vi "Rotation3d_Equals.vi"(9 "other Rotation3d":T1={"Q_quaternion"={"R"=1.0, "V"=[0.0, 0.0, 0.0]}}, 11 "in Rotation3d":T1={"Q_quaternion"={"R"=1.0, "V"=[0.0, 0.0, 0.0]}}) -> (3 "Equals":bool)   [LabVIEW 2019, in "Trajectory_Library.lvlib"]
doc: "Checks equality between this Rotation3d and another object.\n\nParameters:\n\n - IN ROTATION3D -- This rotation3d data structure\n - OTHER ROTATION3D -- The rotation3d to compare.\n\nReturns:\n - Equals -- Returns TRUE if the two rotation3ds are equals."
uses:
  Trajectory_Library.lvlib
  TypeDef/ROTATION3D.ctl
  TypeDef/QUATERNION.ctl
  Quaternion_Get_Vect.vi
  Quaternion_Get_W.vi
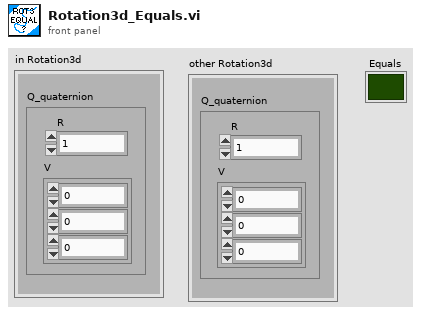
[diagram p1: front panel]
types:
  T1 = typedef "Trajectory_Library.lvlib/ROTATION3D.ctl" = cluster{"Q_quaternion":T2}
  T2 = typedef "Trajectory_Library.lvlib/QUATERNION.ctl" = cluster{"R":dbl, "V":dbl[]}
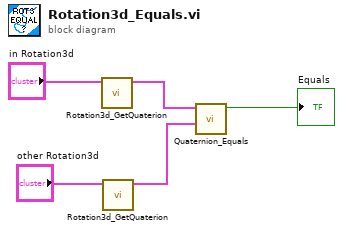
[diagram p0: block diagram]
diagram:
  n1 = call "Rotation3d_GetQuaterion.vi"("in Rotation3d"="in Rotation3d") -> ("out Quaterion"=w3:T2)  [unwired: 10 in]
  n2 = call "Rotation3d_GetQuaterion.vi"("in Rotation3d"="other Rotation3d") -> ("out Quaterion"=w2:T2)  [unwired: 10 in]
  n3 = call "Quaternion_Equals.vi"("Other Quaternion"=w2, "Quaternion"=w3) -> ("Equal"=→"Equals":bool)  [unwired: 9 in]
